vi "Get Acquisition Progress.vi"(10 "series":i32, 11 "acc":i32) -> (1 "function return":u32, 2 "series out":i32, 3 "acc out":i32)   [LabVIEW 2018, in "AndorSDK.lvlib"]
doc: "EXPNETTYPE unsigned int WINAPI GetAcquisitionProgress(long * acc, long * series);"
uses:
  AndorSDK.lvlib
  ATMCD32D.dll
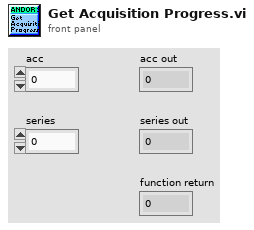
[diagram p1: front panel]
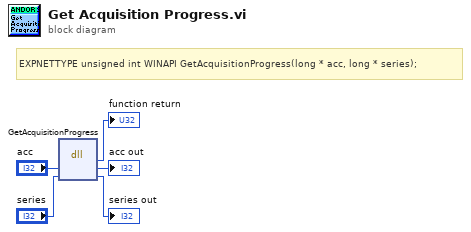
[diagram p0: block diagram]
diagram:
  # "EXPNETTYPE unsigned int WINAPI GetAcquisitionProgress(long * acc, long * series);"
  n1 = dll-call lib="PTH2babs E\nPersönliches02 - Arbeit03-HiwijobsLabviewCodelibANDOR\tAndor SDK\nATMCD32D.*" fn="GetAcquisitionProgress"("acc"="acc", "series"="series") -> (→"function return":u32, "acc"=→"acc out":i32, "series"=→"series out":i32)  [unwired: 3 in, 2 out]
